vi "MessageHandlerProcess.vi"   [LabVIEW 2011]
uses:
  MessageHandlerContext.ctl
  030 - EVENTS/EnumFgvEventCommand.ctl
  030 - EVENTS/03 - ToMessageHandlerProcess/ToMessageHandlerEvent.ctl
  030 - EVENTS/03 - ToMessageHandlerProcess/enumMessageCriticity.ctl
panel:
  # "Message handler process ...\n\nProcessus détaché destiné à l'archivage des messages ..."
types:
  T1 = typedef "MessageHandlerContext.ctl" = cluster{"LogFileName":string, "Message number":i32}
  T2 = typedef "EnumFgvEventCommand.ctl" = enum16{"Setup", "Cleanup", "Get"}
  T3 = typedef "ToMessageHandlerEvent.ctl" = cluster{"date / time":timestamp, "Criticity":T4, "Emitter":string, "Message":string}
  T4 = typedef "enumMessageCriticity.ctl" = enum16{"No error", "Info", "Warning", "Error", "Fatal error"}
  T5 = enum32{"Invalid", "Standard", "Closed", "Hidden", "Minimized", "Maximized"}
  T6 = typedef "EnumToAllProcessesCommand.ctl" = enum16{"Stop all processes", "Autotest"}
  T7 = typedef "ToProcess_EnumCommand.ctl" = enum16{"Show front panel", "Hide front panel"}
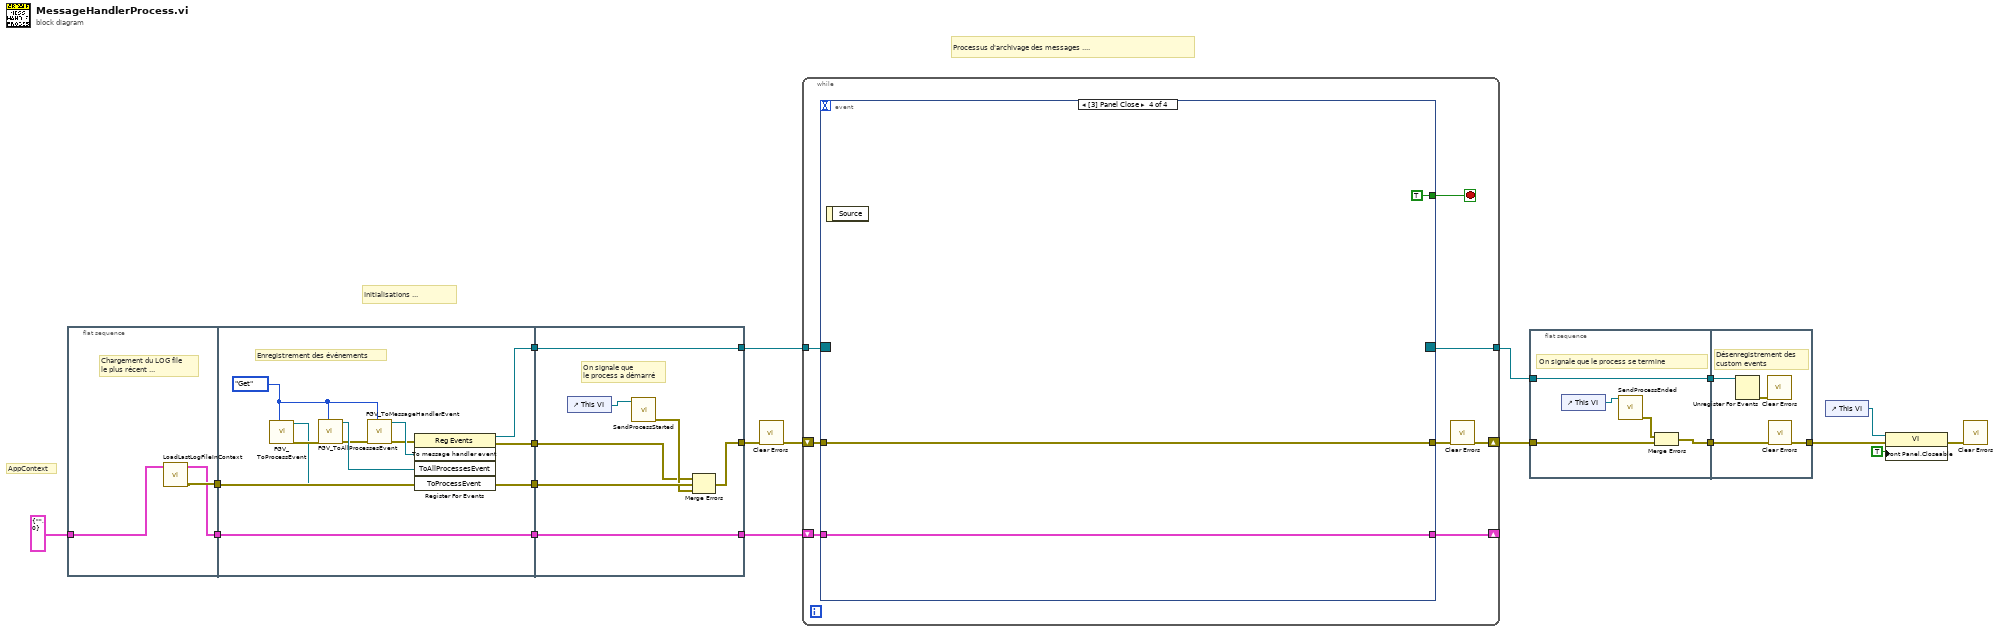
[diagram p0: block diagram]
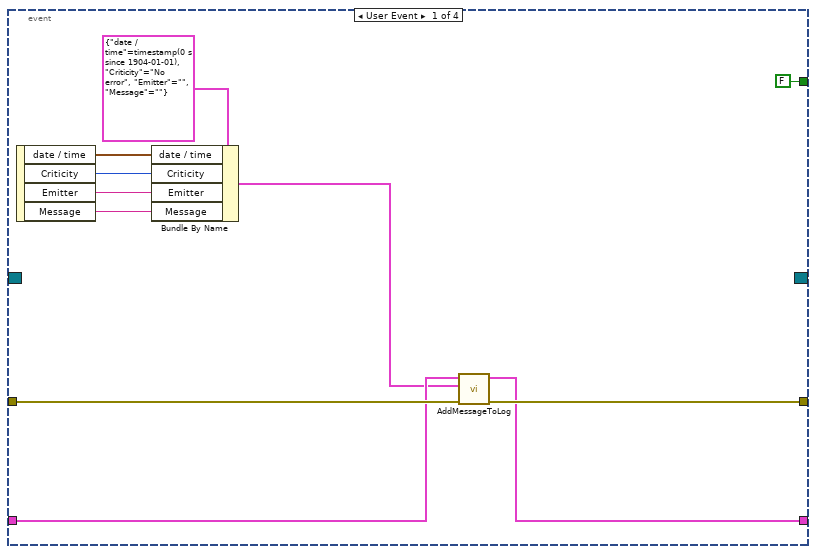
[diagram p2: hidden frame]
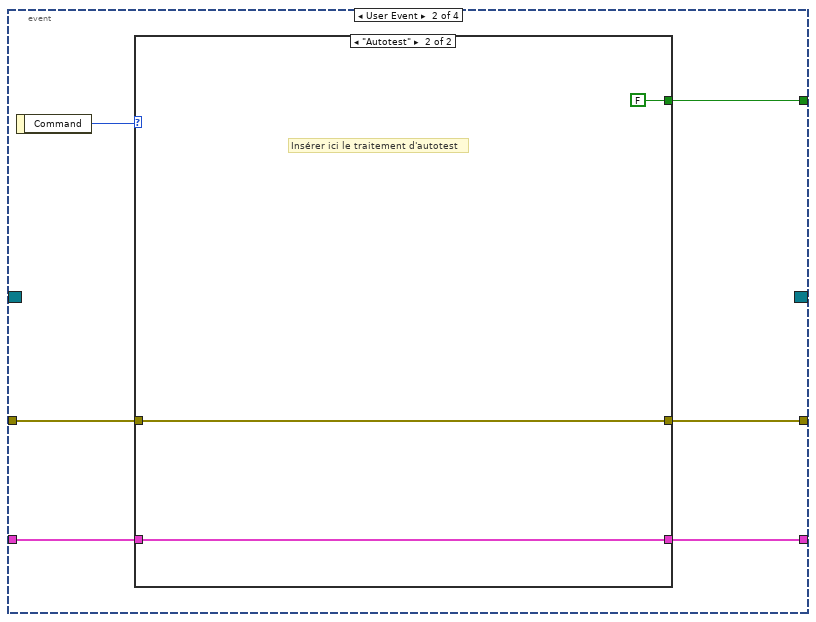
[diagram p3: hidden frame]
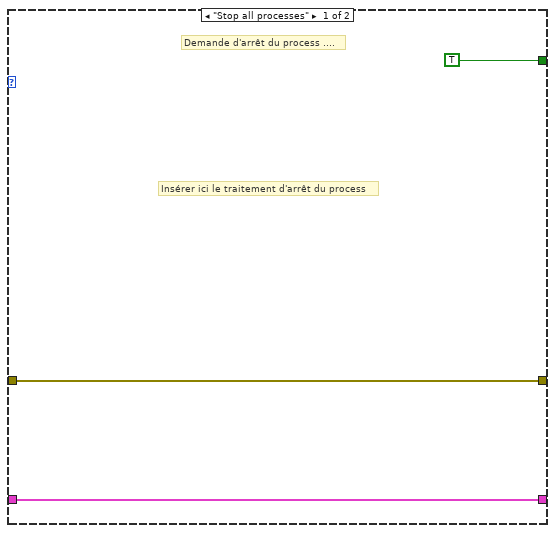
[diagram p4: hidden frame]
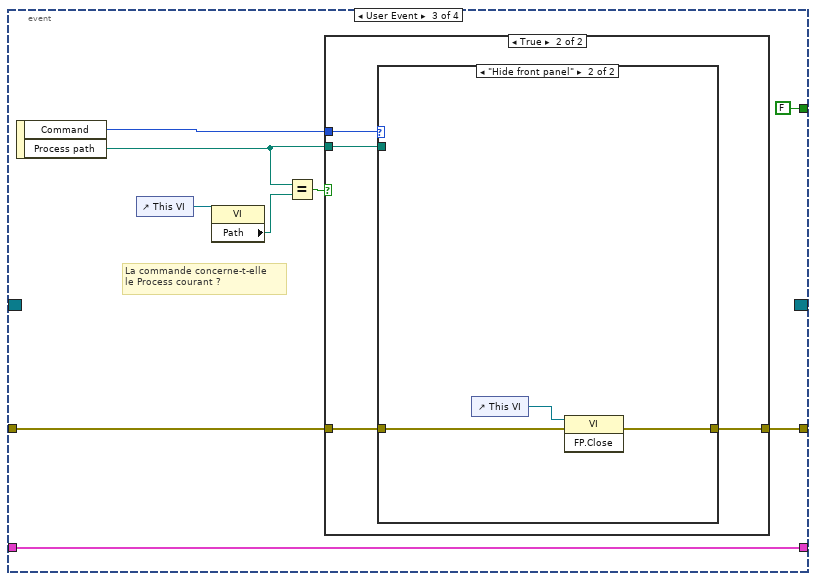
[diagram p5: hidden frame]
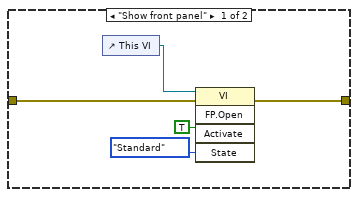
[diagram p7: hidden frame]
diagram:
  # "AppContext"
  # "Initialisations ..."
  # "Processus d'archivage des messages ...."
  n1 = flat-sequence {
    tunnel: [w22] -> w13
    tunnel: T1 {"LogFileName"="", "Message number"=0} ("AppContext") -> [w21]
    tunnel: [w20] -> w11
    tunnel: w13 -> [w33]
    tunnel: [w33] -> w12
    tunnel: w11 -> [w32]
    tunnel: [w32] -> w10
    tunnel: [w27] -> w9
    tunnel: [w26] -> w8
    tunnel: [w39] -> w19
    tunnel: [w36] -> w18
    tunnel: w12 -> [w40]
    tunnel: w10 -> [w38]
    tunnel: [w38] -> w14
    tunnel: w9 -> [w35]
    tunnel: w8 -> [w36]
    frame #0 {
      # "Chargement du LOG file\nle plus récent ..."
      n2 = call "LoadLastLogFileInContext.vi"("AppContextIn"=w21) -> ("error out"=w22:errorcluster, "AppContextOut"=w20:T1)  [unwired: 9 in]
    }
    frame #1 {
      w24 = EnumFgvEventCommand."Get" ("Command")
      # "Enregistrement des événements"
      n3 = call "FGV_ToProcessEvent.vi"("Command"=w24) -> ("error out"=w25:errorcluster, "ToProcessEvent"=w23:refnum<user-event>)  [unwired: 9 in]
      n4 = call "FGV_ToAllProcessesEvent.vi"("Command"=w24, "error in (no error)"=w25) -> ("error out"=w28:errorcluster, "ToAllProcessesEvent"=w31:refnum<user-event>)  [unwired: 8 in]
      n5 = call "FGV_ToMessageHandlerEvent.vi"("Command"=w24, "error in (no error)"=w28) -> ("error out"=w29:errorcluster, "To message handler event"=w30:refnum<user-event>)  [unwired: 8 in]
      n6 = register-events(error in=w29, w30, w31, w23) -> (reference out=w26:refnum<event-registration>, error out=w27:errorcluster)  [unwired: 1 in]
    }
    frame #2 {
      # "On signale que\nle process a démarré"
      n7 = control-ref of="This VI"() -> (w34:refnum<vi>)
      n8 = call "SendProcessStarted.vi"("Process Refnum"=w34) -> ("error out"=w37:errorcluster)  [unwired: 10 in]
      n9 = Merge Errors(w35, w40, w37) -> (w39:errorcluster)
    }
  }
  n10 = call <vilib>:"Clear Errors.vi"("error in (no error)"=w19) -> ("error out"=w7:errorcluster)  [unwired: 6 in]
  n11 = while {
    shift-right: [w44] -> w16
    shift-left: w7 -> [w41]
    tunnel: w18 -> [w47]
    tunnel: [w46] -> w17
    shift-right: [w42] -> _
    shift-left: w14 -> [w43]
    stop <- w45 stop-if-true
    n12 = event shown="[3] Panel Close" {
      selector: w47 -> [_ _ _ _]
      dyn-events: [_ _ _ _] -> w46
      timeout: _ -> [_ _ _ _]
      tunnel: w41 -> [w54 w63 w75 w96]
      tunnel: [w53 w62 w74 w96] -> w48
      tunnel: [FALSE w64 FALSE TRUE] -> w45
      tunnel: w43 -> [w52 w61 w73 w95]
      tunnel: [w51 w60 w73 w95] -> w42
      event User Event {
        n13 = event-data() -> ("date / time"=w58:timestamp, "Criticity"=w57:T4, "Emitter"=w56:string, "Message"=w55:string)  [unwired: 1 in]
        n14 = Bundle By Name(cluster=T3 {"date / time"=timestamp(0 s since 1904-01-01), "Criticity"=enum."No error", "Emitter"="", "Message"=""} ("To message handler event"), "date / time"=w58, "Criticity"=w57, "Emitter"=w56, "Message"=w55) -> (w50:T3)
        n15 = call "AddMessageToLog.vi"("error in (no error)"=w54, "Message"=w50, "AppContextIn"=w52) -> ("error out"=w53:errorcluster, "AppContextOut"=w51:T1)  [unwired: 7 in]
      }
      event User Event {
        n16 = event-data() -> ("Command"=w65:T6)  [unwired: 1 in]
        n17 = case shown="\"Autotest\"" w65 {
          tunnel: [TRUE FALSE] -> w64
          tunnel: w63 -> [w67 w71]
          tunnel: [w67 w71] -> w62
          tunnel: w61 -> [w66 w70]
          tunnel: [w66 w70] -> w60
          frame "Stop all processes" {
            # "Insérer ici le traitement d'arrêt du process"
            # "Demande d'arrêt du process ...."
          }
          frame "Autotest" {
            # "Insérer ici le traitement d'autotest"
          }
        }
      }
      event User Event {
        # "La commande concerne-t-elle\nle Process courant ?"
        n18 = event-data() -> ("Command"=w77:T7, "Process path"=w76:path)  [unwired: 1 in]
        n19 = control-ref of="This VI"() -> (w78:refnum<vi>)
        n20 = property class="VI"(reference=w78) -> ("Path"=w79:path)  [unwired: 1 in, 2 out]
        n21 = Equal?(x=w76, y=w79) -> (x = y?=w80:bool)
        n22 = case shown="True" w80 {
          tunnel: w77 -> [_ w85]
          tunnel: w75 -> [w81 w84]
          tunnel: w76 -> [_ w83]
          tunnel: [w81 w82] -> w74
          frame False {
            # "La commande n'est pas pour ce process !"
          }
          frame True {
            n23 = case shown="\"Hide front panel\"" w85 {
              tunnel: w84 -> [w89 w92]
              tunnel: w83 -> [_ _]
              tunnel: [w88 w91] -> w82
              frame "Show front panel" {
                n24 = control-ref of="This VI"() -> (w90:refnum<vi>)
                n25 = invoke class="VI" method="FP.Open"(reference=w90, error in=w89, "Activate"=TRUE ("Activate?"), "State"=T5."Standard") -> (error out=w88:errorcluster)  [unwired: 1 in, 4 out]
              }
              frame "Hide front panel" {
                n26 = control-ref of="This VI"() -> (w93:refnum<vi>)
                n27 = invoke class="VI" method="FP.Close"(reference=w93, error in=w92) -> (error out=w91:errorcluster)  [unwired: 1 in, 2 out]
              }
            }
          }
        }
      }
      event Panel Close {
        n28 = event-data() -> ()  [unwired: 1 in, 1 out]
      }
    }
    n29 = call <vilib>:"Clear Errors.vi"("error in (no error)"=w48) -> ("error out"=w44:errorcluster)  [unwired: 6 in]
  }
  n30 = flat-sequence {
    tunnel: w16 -> [w99]
    tunnel: w17 -> [w101]
    tunnel: [w101] -> w2
    tunnel: [w98] -> w1
    tunnel: [w102] -> w6
    tunnel: w2 -> [w105]
    tunnel: w1 -> [w103]
    frame #0 {
      # "On signale que le process se termine"
      n31 = control-ref of="This VI"() -> (w97:refnum<vi>)
      n32 = call "SendProcessEnded.vi"("Process Refnum"=w97) -> ("error out"=w100:errorcluster)  [unwired: 10 in]
      n33 = Merge Errors(w100, w99) -> (w98:errorcluster)
    }
    frame #1 {
      # "Désenregistrement des\ncustom events"
      n34 = Unregister For Events(event registration refnum=w105) -> (error out=w104:errorcluster)  [unwired: 1 in]
      n35 = call <vilib>:"Clear Errors.vi"("error in (no error)"=w104) -> ()  [unwired: 6 in, 1 out]
      n36 = call <vilib>:"Clear Errors.vi"("error in (no error)"=w103) -> ("error out"=w102:errorcluster)  [unwired: 6 in]
    }
  }
  n37 = control-ref of="This VI"() -> (w5:refnum<vi>)
  n38 = property class="VI"(reference=w5, error in=w6, "Front Panel.Closeable"=TRUE ("Front Panel Window:Closeable")) -> (error out=w3:errorcluster)  [unwired: 1 out]
  n39 = call <vilib>:"Clear Errors.vi"("error in (no error)"=w3) -> ()  [unwired: 6 in, 1 out]
